vi "CANBusTestTx.vi"(8 "error in (no error)":errorcluster, 9 "value":u8[](array[numeric]), 10 "method":string, 11 "Sequence Context In":refnum<k7>) -> (0 "error out":errorcluster, 2 "status":string)   [LabVIEW 2021]
uses:
  <vilib>/addons/TestStand/_TSUtility.llb/TestStand - Get Property Value (String).vi
  <vilib>/NI/JSON Support for LabVIEW/JSON Value/New JSON Value/New JSON ({}).vi
  <vilib>/NI/JSON Support for LabVIEW/JSON Value/Object/Insert Value/Insert Value (Numeric[]).vi
  <vilib>/NI/NI JSONRPC Server Framework/Classes/Client/Format Client Request (Auto-Increment).vi
  <vilib>/NI/JSON Support for LabVIEW/JSON Value/JSON Value.lvclass
  <vilib>/NI/NI JSONRPC Server Framework/Classes/Client/JSONRPC Client.lvclass
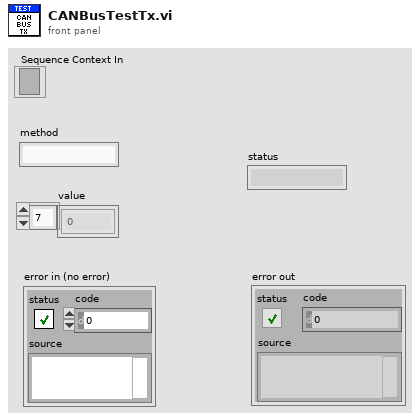
[diagram p1: front panel]
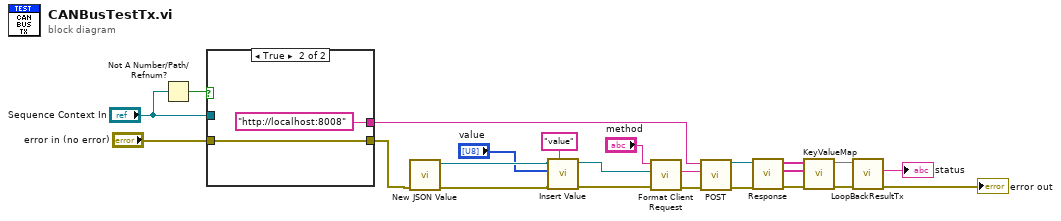
[diagram p0: block diagram]
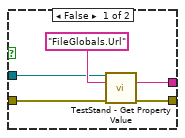
[diagram p2: hidden frame]
diagram:
  n1 = Not A Number/Path/Refnum?(number/path/refnum="Sequence Context In") -> (NaN/Path/Refnum?=w8:bool)
  n2 = case shown="True" w8 {
    tunnel: [w27 "http://localhost:8008" ("Value")] -> w23
    tunnel: [w26 w29] -> w7
    tunnel: "error in (no error)" -> [w25 w29]
    tunnel: "Sequence Context In" -> [w24 _]
    frame False {
      n3 = call-poly <vilib>:"TestStand - Get Property Value.vi"("Sequence Context In"=w24, "Lookup String"="FileGlobals.Url", "error in (no error)"=w25) -> ("Value"=w27:string, "error out"=w26:errorcluster)  [unwired: 10 in, 1 out]
    }
    frame True {
    }
  }
  n4 = call-poly <vilib>:"New JSON Value.vi"("error in (no error)"=w7) -> ("error out"=w6:errorcluster, "JSON Value out"=w5:refnum<class "JSON Value.lvclass">)  [unwired: 9 in]
  n5 = call-poly <vilib>:"Insert Value.vi"("key"="value", "error in (no error)"=w6, "JSON Data in"="value", "JSON Value in"=w5) -> ("error out"=w4:errorcluster, "JSON Value out"=w3:refnum<class "JSON Value.lvclass">)  [unwired: 5 in, 1 out]
  n6 = call-poly <vilib>:"Format Client Request.vi"("error in (no error)"=w4, "JSON Value in"=w3, "method"="method") -> ("error out"=w14:errorcluster, "Request String"=w15:string)  [unwired: 7 in]
  n7 = call "POST.vi"("error in (no error)"=w14, "Request String"=w15, "url"=w23) -> ("error out"=w16:errorcluster, "JSON Value out"=w17:refnum<class "JSON Value.lvclass">)  [unwired: 7 in]
  n8 = call "Response.vi"("error in (no error)"=w16, "JSON Value in"=w17) -> ("error out"=w18:errorcluster, "values"=w20:string[], "keys"=w19:string[])  [unwired: 7 in]
  n9 = call "KeyValueMap.vi"("error in"=w18, "values"=w20, "keys"=w19) -> ("error out"=w11:errorcluster, "map out"=w12:map{string, string})  [unwired: 7 in]
  n10 = call "LoopBackResultTx.vi"("error in (no error)"=w11, "map"=w12) -> ("error out"=→"error out":errorcluster, "status"=→"status":string)  [unwired: 8 in]
